vi "Camera Autofocus.vi"(8 "error in":errorcluster, 10 "Image Size":T1={"H Bin"=1, "V Bin"=1, "Left"=1, "Top"=1, "Right"=512, "Bottom"=512} {"Top" min=4 max=2048 step=4; "Left" min=4 max=2048 step=4; "V Bin" min=1 max=2048 step=4; "H Bin" min=1 max=2048 step=4}, 11 "Display Window Number":i32) -> (0 "error out":errorcluster)   [LabVIEW 2011]
doc: "Aquires a z-stack of images, calculates the goodness-of-focus (GOF) parameter for each image, and returns the stage to the z position with max GOF. Parameters of the autofocusing process are set (and can be adjusted during acquisition) using the Autofocus Globals.vi front panel."
uses:
  ixon camera/image size.ctl
  ixon1024/HAL camera parameters important.ctt
  ixon1024/ixon readout settings.ctl
  ixon1024/andor acquisition mode.ctl
  Stage/Move stage command.ctl
  Autofocus Globals.vi
panel:
  in  "Current z":ext
  out "Goodness of Focus":cluster{ext[], dbl[]}(graph)
  out "Contrast":bool=TRUE
  out "z position":ext(graph)
  # "not for interactive use"
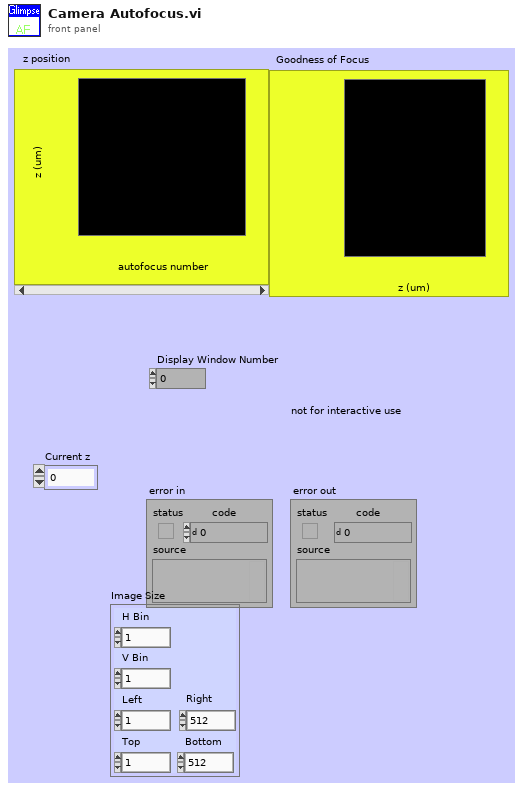
[diagram p1: front panel]
types:
  T1 = typedef "image size.ctl" = cluster{"H Bin":i32, "V Bin":i32, "Left":i32, "Top":i32, "Right":i32, "Bottom":i32}
  T2 = typedef "HAL camera parameters important.ctt" = cluster{"Exposure Time (sec)":sgl, "EM CCD Gain":u16, "Readout Settings":T3, "Image Size":cluster{"H Bin":i32, "V Bin":i32, "Left":i32, "Top":i32, "Right":i32, "Bottom":i32}, "Shutter":i32}
  T3 = typedef "ixon readout settings.ctl" = cluster{"Acquisition Mode":T4, "Pixel Rate":enum16{"EM CCD 10 Mhz 14 bits", "EM CCD 5 Mhz 14 bits", "EM CCD 3 Mhz 14 bits", "EM CCD 1 Mhz 16 bits", "Standard CCD 3 Mhz 14 bits", "Standard CCD 1 Mhz 16 bits"}, "High Capacity?":bool, "V Shift Speed (us/row)":enum16{"0.9 (not reccommended)", "1.7  (not reccommended)", "3.3  (not reccommended)", "6.5", "12.9"}, "V Shift Amplitude":enum16{"normal", "+1", "+2", "+3", "+4"}, "Preamp Gain":enum16{"1.0", "2.4", "5.0"}, "Trigger Mode":u32}
  T4 = typedef "andor acquisition mode.ctl" = enum16{"(do not use)", "Single Scan", "Accumulate", "Kinetics", "Fast Kinetics", "Kinetics Run till Abort", "Frame Transfer", "Frame Transfer Run till Abort", "(do not use) ", "Time Delayed Integration"}
  T5 = typedef "IMAQ Image.ctl" = refnum<image>
  T6 = typedef "Laser type.ctt" = enum16{"Blue 488 nm", "Green 532 nm", "Red 633 nm", "IR 780"}
  T7 = typedef "Move stage command.ctl" = cluster{"dx (um) (0 -> ignore)":ext, "dy (um) (0 -> ignore)":ext, "dz (um) (0 -> ignore)":ext, "Re-center x,y":bool, "Re-center z":bool, "x (um) (-1 -> ignore)":dbl, "y (um) (-1 -> ignore)":dbl, "z (um) (-1 -> ignore)":dbl}
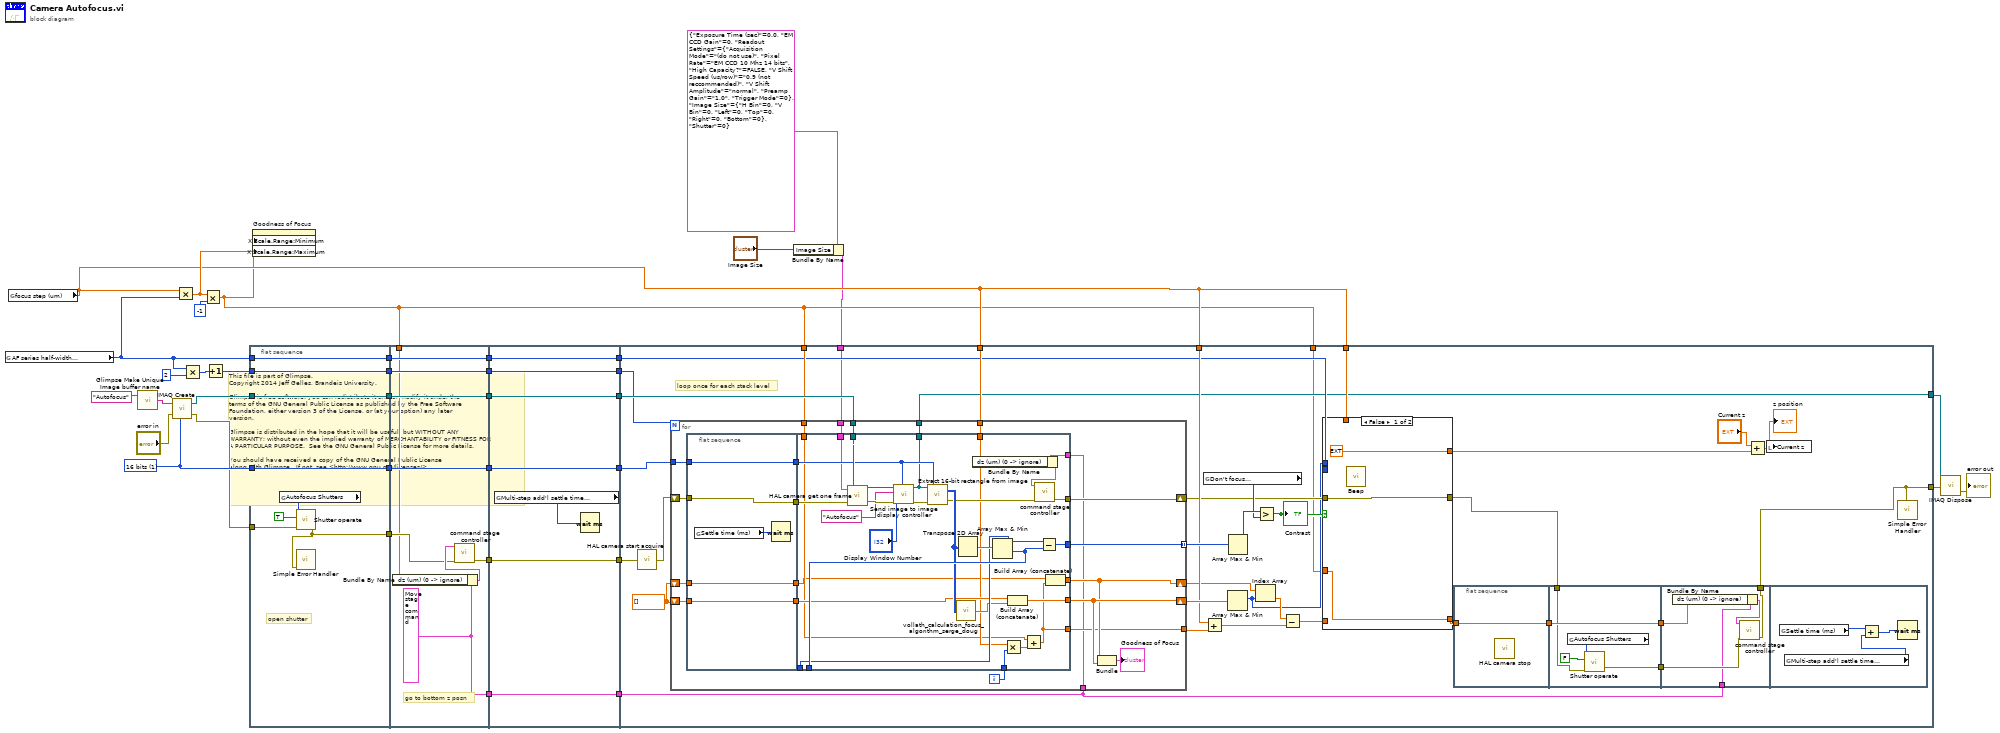
[diagram p0: block diagram]
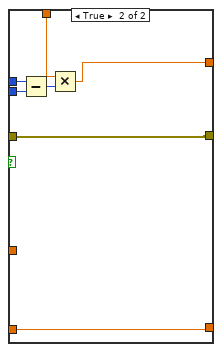
[diagram p2: hidden frame]
diagram:
  w31 = u32 1 items=["8 bits", "16 bits", "Float", "Complex", "RGB", "HSL"] ("pixel depth")
  # "This file is part of Glimpse. \nCopyright 2014 Jeff Gelles, Brandeis University.    \n\nGlimpse is free software: you can redistribute it and/or modify it under the \nterms of the GNU General Public License as published by the Free Software \nFoundation, either version 3 of the License, or (at your option) any later \nversion.\n\nGlimpse is distributed in the hope that it will be useful, but WITHOUT ANY \nWARRANTY; without even the implied warranty of MERCHANTABILITY or FITNESS FOR \nA PARTICULAR PURPOSE.  See the GNU General Public License for more details.\n\nYou should have received a copy of the GNU General Public License\nalong with Glimpse.  If not, see <http://www.gnu.org/licenses/>."
  n1 = global read "Autofocus Globals.vi" "AF series half-width\n (steps)"() -> (w30:u16)
  n2 = global read "Autofocus Globals.vi" "focus step (um)"() -> (w22:ext)
  n3 = call "Glimpse Make Unique Image buffer name.vi"("Buffer  base name"="Autofocus" ("Image Name")) -> ("Image Name"=w18:string)  [unwired: 1 out]
  n4 = call "IMAQ Create"("Image Name"=w18, "Image Type"=w31, "error in (no error)"="error in") -> ("New Image"=w36:T5, "error out"=w23:errorcluster)  [unwired: 1 in, 1 out]
  n5 = Multiply(x=w22, y=w30) -> (x*y=w24:ext)
  n6 = Multiply(x=w30, y=i16 2) -> (x*y=w34:u16)
  n7 = Multiply(x=w24, y=i16 -1) -> (x*y=w6:ext)
  n8 = Increment(x=w34) -> (x+1=w32:u16)
  n9 = flat-sequence {
    tunnel: w30 -> [w42]
    tunnel: w32 -> [w43]
    tunnel: w31 -> [w44]
    tunnel: w36 -> [w45]
    tunnel: [w45] -> w29
    tunnel: [w44] -> w28
    tunnel: [w43] -> w27
    tunnel: [w42] -> w26
    tunnel: w23 -> [w40]
    tunnel: [w38] -> w25
    tunnel: w29 -> [w54]
    tunnel: [w54] -> w16
    tunnel: w28 -> [w53]
    tunnel: [w53] -> w14
    tunnel: w27 -> [w52]
    tunnel: [w52] -> w12
    tunnel: w26 -> [w51]
    tunnel: [w51] -> w10
    tunnel: w6 -> [w47]
    tunnel: w25 -> [w49]
    tunnel: [w48] -> w8
    tunnel: [w46] -> w4
    tunnel: w16 -> [w61]
    tunnel: [w61] -> w15
    tunnel: w14 -> [w60]
    tunnel: [w60] -> w13
    tunnel: w12 -> [w59]
    tunnel: [w59] -> w11
    tunnel: w10 -> [w58]
    tunnel: [w58] -> w9
    tunnel: w8 -> [w57]
    tunnel: [w57] -> w7
    tunnel: [w55] -> w5
    tunnel: w4 -> [w55]
    tunnel: w15 -> [w97]
    tunnel: w13 -> [w96]
    tunnel: w11 -> [w95]
    tunnel: w9 -> [w76]
    tunnel: w7 -> [w92]
    tunnel: w22 -> [w90]
    tunnel: w6 -> [w88]
    tunnel: w22 -> [w83]
    tunnel: w22 -> [w75]
    tunnel: [w69] -> w21
    tunnel: [w71] -> w19
    tunnel: w6 -> [w68]
    tunnel: w5 -> [w63]
    tunnel: w1 -> [w62]
    frame #0 {
      # "open shutter"
      n10 = global read "Autofocus Globals.vi" "Autofocus Shutters"() -> (w39:T6[])
      n11 = call "Shutter operate.vi"("Shutters"=w39, 2:TRUE ("Data to Write"), "error in"=w40) -> ("error out"=w38:errorcluster)  [unwired: 5 out]
      n12 = call <vilib>:"Simple Error Handler.vi"("error in (no error)"=w38) -> ()  [unwired: 1 in, 8 out]
    }
    frame #1 {
      w46 = T7 {"dx (um) (0 -> ignore)"=0.0, "dy (um) (0 -> ignore)"=0.0, "dz (um) (0 -> ignore)"=0.0, "Re-center x,y"=FALSE, "Re-center z"=FALSE, "x (um) (-1 -> ignore)"=-1.0, "y (um) (-1 -> ignore)"=-1.0, "z (um) (-1 -> ignore)"=-1.0} ("command")
      # "go to bottom z posn"
      n13 = Bundle By Name(cluster=w46, "dz (um) (0 -> ignore)"=w47) -> (w50:T7)
      n14 = call "command stage controller.vi"("command"=w50, "error in (no error)"=w49) -> ("error out"=w48:errorcluster)  [unwired: 6 out]
    }
    frame #2 {
      n15 = global read "Autofocus Globals.vi" "Multi-step add'l settle time\n(ms)"() -> (w56:u16)
      n16 = Wait (ms)(milliseconds to wait=w56) -> ()  [unwired: 1 out]
    }
    frame #3 {
      w89 = dbl[] []
      # "loop once for each stack level"
      n17 = call "HAL camera start acquire.vi"("error in"=w92) -> ("error out"=w91:errorcluster)
      n18 = for {
        N: w95 -> [_]
        shift-right: [w135] -> w78
        shift-left: w91 -> [w137]
        tunnel: w97 -> [w139]
        tunnel: w96 -> [w142]
        tunnel: [w141] -> w93 mode=indexing
        tunnel: w90 -> [w136]
        shift-right: [w127] -> w86
        shift-left: w89 -> [w134]
        shift-right: [w126] -> w81
        shift-left: w89 -> [w129]
        tunnel: w88 -> [w131]
        tunnel: [w125] -> w84
        tunnel: [w124] -> w71
        tunnel: w63 -> [w123]
        tunnel: w62 -> [w122]
        i -> [w132]
        n19 = flat-sequence {
          tunnel: w142 -> [w146]
          tunnel: [w146] -> w140
          tunnel: w137 -> [w145]
          tunnel: [w145] -> w138
          tunnel: w134 -> [w144]
          tunnel: [w144] -> w133
          tunnel: [w143] -> w130
          tunnel: w129 -> [w143]
          tunnel: [w176] -> w141
          tunnel: w140 -> [w166]
          tunnel: [w174] -> _
          tunnel: [w173] -> _
          tunnel: w139 -> [w172]
          tunnel: w138 -> [w171]
          tunnel: w136 -> [w156]
          tunnel: [w161] -> w135
          tunnel: [w159] -> w127
          tunnel: w133 -> [w158]
          tunnel: w132 -> [w157]
          tunnel: w131 -> [w154]
          tunnel: w130 -> [w153]
          tunnel: [w152] -> w126
          tunnel: [w151] -> w125
          tunnel: [w150] -> w124
          tunnel: w123 -> [w149]
          tunnel: w122 -> [w148]
          frame #0 {
            n20 = global read "Autofocus Globals.vi" "Settle time (ms)"() -> (w147:u16)
            n21 = Wait (ms)(milliseconds to wait=w147) -> ()  [unwired: 1 out]
          }
          frame #1 {
            n22 = call "HAL camera get one frame.vi"("error in"=w171, "New Image"=w172, "Camera Parameters (important)"=w148) -> ("error out"=w169:errorcluster, "Image Out"=w170:T5)
            n23 = call "Send image to image display controller.vi"("Image"=w170, "Window Title"="Autofocus", "Window Number"="Display Window Number", "error in"=w169, "Image Type"=w166) -> ("Image Out"=w150:T5, "error out"=w165:errorcluster)  [unwired: 2 in, 2 out]
            n24 = call "Extract 16-bit rectangle from image.vi"("error in"=w165, "Image pixel depth"=w166, "Image in"=w150) -> ("error out"=w162:errorcluster, "Image Pixels (I16)"=w164:i16[][])  [unwired: 1 in]
            n25 = call "vollath_calculation_focus_algorithm_serge_doug.vi"("Array"=w164) -> ("VollVal"=w160:dbl)
            n26 = Transpose 2D Array(2D array=w164) -> (transposed array=w175:i16[][])
            n27 = Bundle By Name(cluster=w149, "dz (um) (0 -> ignore)"=w156) -> (w163:T7)
            n28 = Array Max & Min(array=w175) -> (max value=w173:i16, min value=w174:i16)  [unwired: 2 out]
            n29 = Multiply(x=w156, y=w157) -> (x*y=w155:ext)
            n30 = Build Array (concatenate)(w158, w160) -> (w159:dbl[])
            n31 = Add(x=w154, y=w155) -> (x+y=w151:ext)
            n32 = call "command stage controller.vi"("command"=w163, "error in (no error)"=w162) -> ("error out"=w161:errorcluster)  [unwired: 6 out]
            n33 = Subtract(x=w173, y=w174) -> (x-y=w176:i16)
            n34 = Build Array (concatenate)(w153, w151) -> (w152:ext[])
          }
        }
        n35 = Bundle(w126, w127) -> (→"Goodness of Focus":cluster{ext[], dbl[]})  [unwired: 1 out]
      }
      n36 = global read "Autofocus Globals.vi" "Don't focus\nif contrast <"() -> (w87:i16)
      n37 = Add(x=w83, y=w84) -> (x+y=w82:ext)
      n38 = Array Max & Min(array=w86) -> (max index (indices)=w77:i32)  [unwired: 3 out]
      n39 = Array Max & Min(array=w93) -> (max value=w94:i16)  [unwired: 3 out]
      n40 = Index Array(array=w81, index=w77) -> (element=w80:ext)
      n41 = Greater?(x=w94, y=w87) -> (0:w85:bool)
      "Contrast" <- w85
      n42 = Subtract(x=w80, y=w82) -> (x-y=w79:ext)
      n43 = case shown="False" w85 {
        tunnel: w79 -> [_ w115]
        tunnel: w78 -> [w113 w116]
        tunnel: w77 -> [_ w121]
        tunnel: w76 -> [_ w120]
        tunnel: w75 -> [_ w118]
        tunnel: [w113 w116] -> w65
        tunnel: [ext 0.0 w117] -> w73
        tunnel: [w112 w115] -> w70
        tunnel: w68 -> [w112 _]
        frame False {
          n44 = call <vilib>:"Beep.vi"() -> ()  [unwired: 3 in, 9 out]
        }
        frame True {
          n45 = Subtract(x=w121, y=w120) -> (x-y=w119:i32)
          n46 = Multiply(x=w118, y=w119) -> (x*y=w117:ext)
        }
      }
      n47 = flat-sequence {
        tunnel: w70 -> [w98]
        tunnel: [w98] -> w66
        tunnel: [w103] -> w67
        tunnel: w66 -> [w103]
        tunnel: w65 -> [w100]
        tunnel: [w99] -> w64
        tunnel: [w106] -> w69
        tunnel: w67 -> [w107]
        tunnel: w64 -> [w105]
        tunnel: w63 -> [w104]
        frame #0 {
          n48 = call "HAL camera stop.vi"() -> ()  [unwired: 1 out]
        }
        frame #1 {
          n49 = global read "Autofocus Globals.vi" "Autofocus Shutters"() -> (w102:T6[])
          n50 = call "Shutter operate.vi"("Shutters"=w102, 2:FALSE ("Data to Write"), "error in"=w100) -> ("error out"=w99:errorcluster)  [unwired: 5 out]
        }
        frame #2 {
          n51 = Bundle By Name(cluster=w104, "dz (um) (0 -> ignore)"=w107) -> (w108:T7)
          n52 = call "command stage controller.vi"("command"=w108, "error in (no error)"=w105) -> ("error out"=w106:errorcluster)  [unwired: 6 out]
        }
        frame #3 {
          n53 = global read "Autofocus Globals.vi" "Settle time (ms)"() -> (w111:u16)
          n54 = global read "Autofocus Globals.vi" "Multi-step add'l settle time\n(ms)"() -> (w109:u16)
          n55 = Add(x=w111, y=w109) -> (x+y=w110:u16)
          n56 = Wait (ms)(milliseconds to wait=w110) -> ()  [unwired: 1 out]
        }
      }
      n57 = Add(x="Current z", y=w73) -> (x+y=w72:ext)
      "z position" <- w72
      n58 = local write "Current z"(w72) -> ()
      n59 = call <vilib>:"Simple Error Handler.vi"("error in (no error)"=w69) -> ()  [unwired: 1 in, 8 out]
    }
  }
  n60 = property on="Goodness of Focus" class="XYGraph (strict)"("X Scale.Range:Minimum"=w6, "X Scale.Range:Maximum"=w24) -> ()  [unwired: 2 in, 2 out]
  n61 = Bundle By Name(cluster=T2 {"Exposure Time (sec)"=0.0, "EM CCD Gain"=0, "Readout Settings"={"Acquisition Mode"=enum."(do not use)", "Pixel Rate"=enum."EM CCD 10 Mhz 14 bits", "High Capacity?"=FALSE, "V Shift Speed (us/row)"=enum."0.9 (not reccommended)", "V Shift Amplitude"=enum."normal", "Preamp Gain"=enum."1.0", "Trigger Mode"=0}, "Image Size"={"H Bin"=0, "V Bin"=0, "Left"=0, "Top"=0, "Right"=0, "Bottom"=0}, "Shutter"=0} ("Camera Parameters (important)"), "Image Size"="Image Size") -> (w1:T2)
  n62 = call "IMAQ Dispose"("Image"=w19, "error in (no error)"=w21) -> ("error out"=→"error out":errorcluster)  [unwired: 1 in, 3 out]
